vi "Finding_Problem_Dots-3.vi"(3 "error IN":errorcluster, 5 "[IN] Frame-to-frame displ":dbl[][](array[numeric])) -> (0 "error OUT":errorcluster, 2 "[OUT] Dot matrix":i16[][](array[numeric]))   [LabVIEW 2013]
doc: "SubVI searches and highlight the problem displacements for further tracks separation"
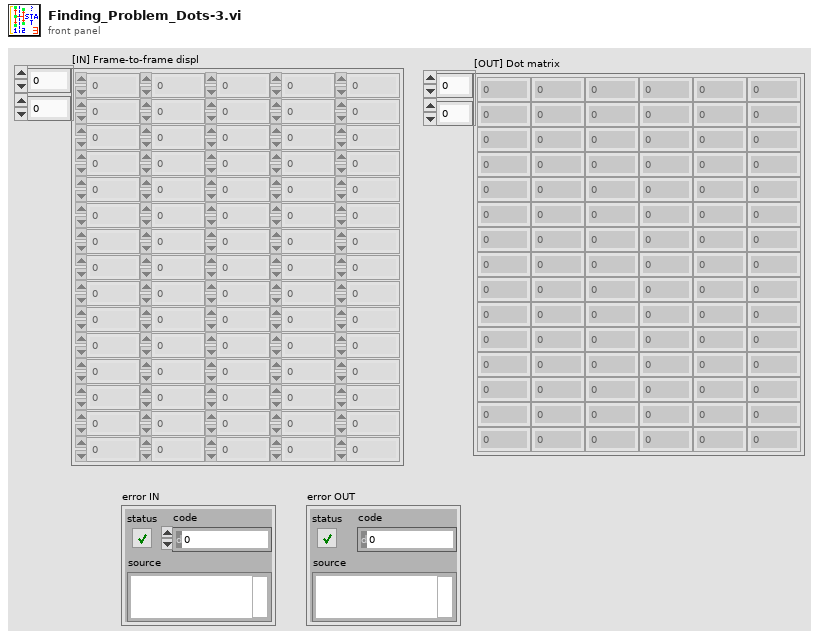
[diagram p1: front panel]
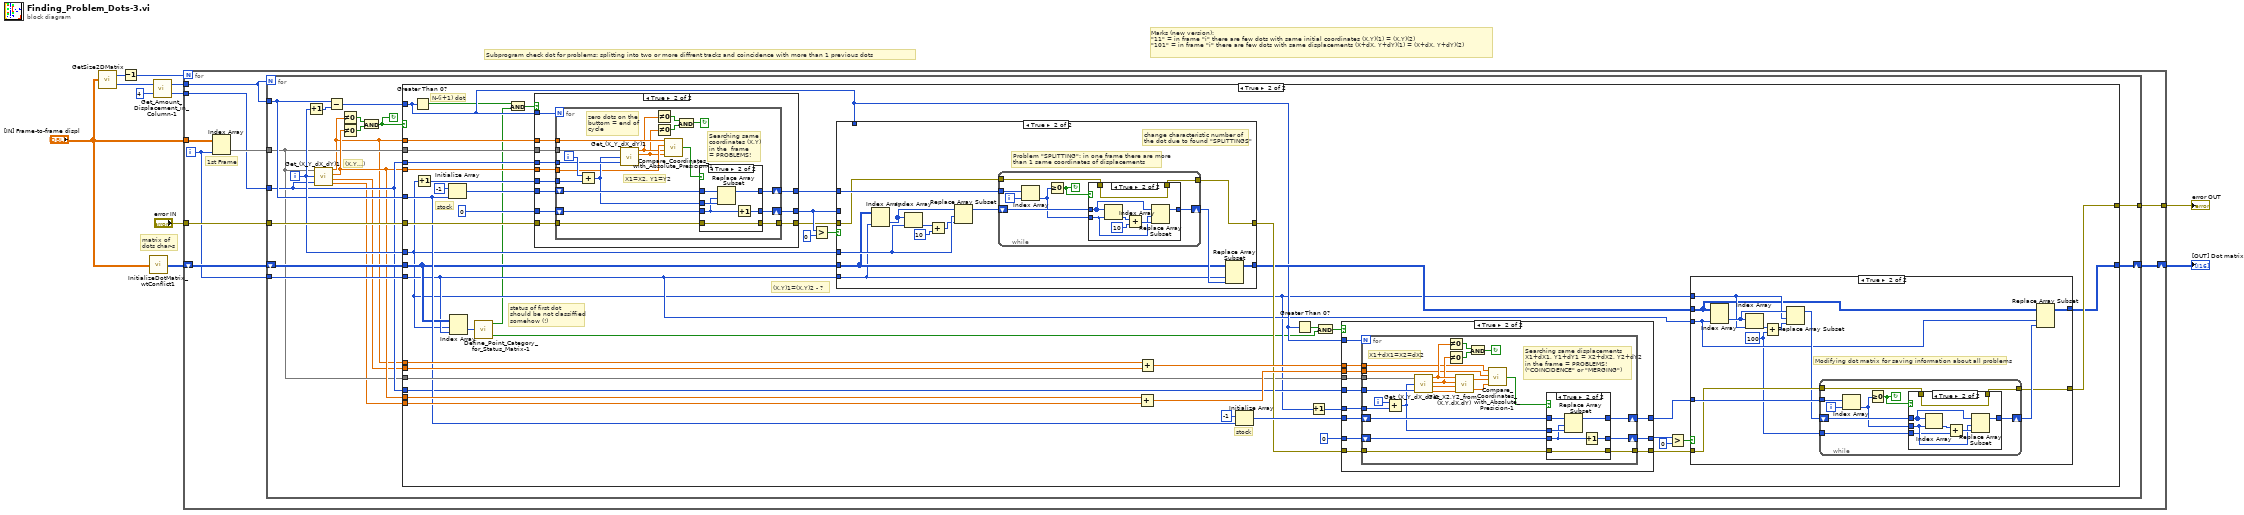
[diagram p0: block diagram]
diagram:
  # "Marks (new version): \n\"11\" = in frame \"i\" there are few dots with same initial coordinates (X,Y)(1) = (X,Y)(2)\n\"101\" = in frame \"i\" there are few dots with same displacements (X+dX, Y+dY)(1) = (X+dX, Y+dY)(2)"
  # "matrix of\ndots char-s"
  # "Subprogram check dot for problems: splitting into two or more diffrent tracks and coincidence with more than 1 previous dots"
  n1 = call "GetSize2DMatrix.vi"("Array IN (2D)"="[IN] Frame-to-frame displ") -> ("# Cols"=w9:i32, "# Rows"=w4:i32)
  n2 = Decrement(x=w9) -> (x-1=w11:i32)
  n3 = call "InitializeDotMatrix_wtConflict1.vi"("Frame-to-frame displ"="[IN] Frame-to-frame displ") -> ("Dot matrix"=w8:i16[][])
  n4 = call "Get_Amount_Displacement_in_Column-1.vi"("multiplier"=4 ("y"), "# Rows"=w4) -> ("multiplier out"=w1:i32, "Displ amount"=w2:i32)
  n5 = for {
    N: w11 -> [_]
    tunnel: "error IN" -> [w20]
    tunnel: [w19] -> w7
    shift-right: [w14] -> w6
    shift-left: w8 -> [w16]
    tunnel: "[IN] Frame-to-frame displ" -> [w17]
    tunnel: w2 -> [w13]
    tunnel: w1 -> [w12]
    i -> [w15]
    # "1st Frame"
    n6 = Index Array(array=w17, index (col)=w15) -> (element=w18:dbl[])  [unwired: 1 in]
    n7 = for {
      N: w13 -> [_]
      tunnel: w12 -> [w26]
      tunnel: w20 -> [w36]
      tunnel: [w35] -> w19
      tunnel: w18 -> [w24]
      tunnel: w13 -> [w30]
      shift-right: [w27] -> w14
      shift-left: w16 -> [w29]
      tunnel: w15 -> [w28]
      i -> [w33]
      stop <- w34 continue-if-true
      # "(X,Y...)"
      n8 = Increment(x=w33) -> (x+1=w32:i32)
      n9 = call "Get_(X_Y_dX_dY)1.vi"("(X,Y,dX,dY)"=w24, "index"=w33, "multiplier"=w26) -> ("X"=w21:dbl, "Y"=w25:dbl, "dX"=w23:dbl, "dY"=w22:dbl)
      n10 = Subtract(x=w30, y=w32) -> (x-y=w31:i32)
      n11 = Not Equal To 0?(x=w21) -> (x != 0?=w38:bool)
      n12 = Not Equal To 0?(x=w25) -> (x != 0?=w37:bool)
      n13 = And(x=w38, y=w37) -> (x .and. y?=w34:bool)
      n14 = case shown="True" w34 {
        tunnel: w21 -> [_ w84]
        tunnel: w25 -> [_ w82]
        tunnel: w36 -> [w40 w77]
        tunnel: [w40 w52] -> w35
        tunnel: w33 -> [_ w46]
        tunnel: w31 -> [_ w60]
        tunnel: w24 -> [_ w85]
        tunnel: w26 -> [_ w83]
        tunnel: w30 -> [_ w54]
        tunnel: w29 -> [w39 w48]
        tunnel: w28 -> [_ w47]
        tunnel: [w39 w51] -> w27
        tunnel: w26 -> [_ w53]
        tunnel: w21 -> [_ w59]
        tunnel: w25 -> [_ w57]
        tunnel: w24 -> [_ w55]
        tunnel: w23 -> [_ w58]
        tunnel: w22 -> [_ w56]
        frame False {
        }
        frame True {
          # "status of first dot\nshould be not classiffied\nsomehow (!)"
          # "stock"
          # "(X,Y)1=(X,Y)2 - ?"
          # "stock"
          # "N-(i+1) dot"
          n15 = Greater Than 0?(x=w60) -> (x > 0?=w50:bool)
          n16 = Increment(x=w46) -> (x+1=w81:i32)
          n17 = Initialize Array(-1 ("element"), w54) -> (w79:i32[])
          n18 = Index Array(array=w48, index (row)=w46, index (col)=w47) -> (element=w45:i16)
          n19 = call "Define_Point_Category_for_Status_Matrix-1.vi"("[IN] Summarized\npoint status"=w45) -> ("[OUT] Point isn't \nlabeled with \"10\""=w44:bool, "[OUT] Point isn't \nlabeled with \"100\""=w41:bool)  [unwired: 1 out]
          n20 = And(x=w50, y=w44) -> (x .and. y?=w49:bool)
          n21 = case shown="True" w49 {
            tunnel: w60 -> [_ w182]
            tunnel: w85 -> [_ w181]
            tunnel: w84 -> [_ w180]
            tunnel: w82 -> [_ w179]
            tunnel: w83 -> [_ w178]
            tunnel: w81 -> [_ w177]
            tunnel: [w170 w176] -> w74
            tunnel: [w169 w175] -> w76
            tunnel: w79 -> [w170 w174]
            tunnel: 0 -> [w169 w173]
            tunnel: w77 -> [w168 w172]
            tunnel: [w168 w171] -> w75
            frame False {
            }
            frame True {
              n22 = for {
                N: w182 -> [_]
                tunnel: w178 -> [w192]
                tunnel: w181 -> [w201]
                tunnel: w180 -> [w186]
                tunnel: w179 -> [w185]
                shift-right: [w196] -> w175
                shift-left: w173 -> [w197]
                tunnel: w177 -> [w194]
                shift-right: [w191] -> w176
                shift-left: w174 -> [w193]
                tunnel: w172 -> [w190]
                tunnel: [w189] -> w171
                i -> [w195]
                stop <- w198 continue-if-true
                # "zero dots on the\nbuttom = end of\ncycle"
                # "X1=X2, Y1=Y2"
                # "Searching same \ncoordinates (X,Y) \nin the  frame \n= PROBLEMS!"
                n23 = Add(x=w195, y=w194) -> (x+y=w188:i32)
                n24 = call "Get_(X_Y_dX_dY)1.vi"("(X,Y,dX,dY)"=w201, "index"=w188, "multiplier"=w192) -> ("X"=w184:dbl, "Y"=w183:dbl)  [unwired: 2 out]
                n25 = Not Equal To 0?(x=w184) -> (x != 0?=w200:bool)
                n26 = Not Equal To 0?(x=w183) -> (x != 0?=w199:bool)
                n27 = call "Compare_Coordinates_with_Absolute_Presicion-1.vi"("X 1"=w186, "Y 1"=w185, "X 2"=w184, "Y 2"=w183) -> ("[OUT] Same coordinates?"=w187:bool)  [unwired: 1 in]
                n28 = And(x=w200, y=w199) -> (x .and. y?=w198:bool)
                n29 = case shown="True" w187 {
                  tunnel: w197 -> [w204 w207]
                  tunnel: [w204 w206] -> w196
                  tunnel: w193 -> [w202 w210]
                  tunnel: w188 -> [_ w209]
                  tunnel: [w202 w208] -> w191
                  tunnel: [w203 w205] -> w189
                  tunnel: w190 -> [w203 w205]
                  frame False {
                  }
                  frame True {
                    n30 = Replace Array Subset(array=w210, new element=w209, index=w207) -> (w208:i32[])
                    n31 = Increment(x=w207) -> (x+1=w206:i32)
                  }
                }
              }
            }
          }
          n32 = Greater?(x=w76, y=0) -> (0:w86:bool)
          n33 = case shown="True" w86 {
            tunnel: w74 -> [_ w224]
            tunnel: w76 -> [_ _]
            tunnel: w75 -> [w212 w217]
            tunnel: w46 -> [_ w225]
            tunnel: [w212 w213] -> w62
            tunnel: w48 -> [w211 w216]
            tunnel: w47 -> [_ w215]
            tunnel: [w211 w214] -> w61
            tunnel: w60 -> [_ _]
            frame False {
            }
            frame True {
              # "change characteristic number of \nthe dot due to found \"SPLITTINGS\""
              # "Problem \"SPLITTING\": in one frame there are more \nthan 1 same coordinates of displacements"
              n34 = Index Array(array=w216, index (col)=w215) -> (element=w223:i16[])  [unwired: 1 in]
              n35 = Index Array(array=w223, index=w225) -> (element=w221:i16)
              n36 = Add(x=w221, y=i16 10) -> (x+y=w219:i16)
              n37 = Replace Array Subset(array=w223, new element=w219, index=w225) -> (w218:i16[])
              n38 = while {
                tunnel: w224 -> [w233]
                shift-right: [w228] -> w222
                shift-left: w218 -> [w230]
                tunnel: w217 -> [w227]
                tunnel: [w226] -> w213
                i -> [w232]
                stop <- w231 continue-if-true
                n39 = Index Array(array=w233, index=w232) -> (element=w229:i32)
                n40 = Greater Or Equal To 0?(x=w229) -> (x >= 0?=w231:bool)
                n41 = case shown="True" w231 {
                  tunnel: w230 -> [w235 w239]
                  tunnel: w229 -> [_ w238]
                  tunnel: [w235 w237] -> w228
                  tunnel: w227 -> [w234 w236]
                  tunnel: [w234 w236] -> w226
                  frame False {
                  }
                  frame True {
                    n42 = Index Array(array=w239, index=w238) -> (element=w241:i16)
                    n43 = Add(x=w241, y=i16 10) -> (x+y=w240:i16)
                    n44 = Replace Array Subset(array=w239, new element=w240, index=w238) -> (w237:i16[])
                  }
                }
              }
              n45 = Replace Array Subset(array=w216, new element=w222, index (col)=w215) -> (w214:i16[][])  [unwired: 1 in]
            }
          }
          n46 = Add(x=w57, y=w56) -> (x+y=w64:dbl)
          n47 = Add(x=w59, y=w58) -> (x+y=w63:dbl)
          n48 = Initialize Array(-1 ("element"), w54) -> (w68:i32[])
          n49 = Greater Than 0?(x=w60) -> (x > 0?=w43:bool)
          n50 = Increment(x=w46) -> (x+1=w65:i32)
          n51 = And(x=w43, y=w41) -> (x .and. y?=w42:bool)
          n52 = case shown="True" w42 {
            tunnel: w60 -> [_ w135]
            tunnel: w55 -> [_ w134]
            tunnel: w63 -> [_ w133]
            tunnel: w64 -> [_ w132]
            tunnel: w53 -> [_ w131]
            tunnel: w65 -> [_ w130]
            tunnel: [w123 w129] -> w73
            tunnel: [w122 w128] -> w70
            tunnel: w68 -> [w123 w127]
            tunnel: 0 -> [w122 w126]
            tunnel: w62 -> [w121 w125]
            tunnel: [w121 w124] -> w72
            frame False {
            }
            frame True {
              n53 = for {
                N: w135 -> [_]
                tunnel: w131 -> [w149]
                tunnel: w134 -> [w158]
                tunnel: w133 -> [w138]
                tunnel: w132 -> [w137]
                shift-right: [w153] -> w128
                shift-left: w126 -> [w154]
                tunnel: w130 -> [w151]
                shift-right: [w148] -> w129
                shift-left: w127 -> [w150]
                tunnel: w125 -> [w147]
                tunnel: [w146] -> w124
                i -> [w152]
                stop <- w155 continue-if-true
                # "X1+dX1=X2=dX2"
                # "Searching same displacements \nX1+dX1, Y1+dY1 = X2+dX2, Y2+dY2\nin the frame = PROBLEMS! (\"COINCIDENCE\" or \"MERGING\")"
                n54 = Add(x=w152, y=w151) -> (x+y=w145:i32)
                n55 = call "Get_(X_Y_dX_dY)1.vi"("(X,Y,dX,dY)"=w158, "index"=w145, "multiplier"=w149) -> ("X"=w144:dbl, "Y"=w143:dbl, "dX"=w142:dbl, "dY"=w141:dbl)
                n56 = Not Equal To 0?(x=w144) -> (x != 0?=w157:bool)
                n57 = Not Equal To 0?(x=w143) -> (x != 0?=w156:bool)
                n58 = call "Get_X2,Y2_from_(X,Y,dX,dY).vi"("dY"=w141, "dX"=w142, "Y1"=w143, "X1"=w144) -> ("Y2 = (Y1+dY)"=w139:dbl, "X2 = (X1+dX)"=w140:dbl)
                n59 = And(x=w157, y=w156) -> (x .and. y?=w155:bool)
                n60 = call "Compare_Coordinates_with_Absolute_Presicion-1.vi"("X 1"=w138, "Y 1"=w137, "X 2"=w140, "Y 2"=w139) -> ("[OUT] Same coordinates?"=w136:bool)  [unwired: 1 in]
                n61 = case shown="True" w136 {
                  tunnel: w154 -> [w161 w164]
                  tunnel: [w161 w163] -> w153
                  tunnel: w150 -> [w159 w167]
                  tunnel: w145 -> [_ w166]
                  tunnel: [w159 w165] -> w148
                  tunnel: [w160 w162] -> w146
                  tunnel: w147 -> [w160 w162]
                  frame False {
                  }
                  frame True {
                    n62 = Replace Array Subset(array=w167, new element=w166, index=w164) -> (w165:i32[])
                    n63 = Increment(x=w164) -> (x+1=w163:i32)
                  }
                }
              }
            }
          }
          n64 = Greater?(x=w70, y=0) -> (0:w71:bool)
          n65 = case shown="True" w71 {
            tunnel: w61 -> [w88 w95]
            tunnel: w47 -> [_ w94]
            tunnel: w46 -> [_ w99]
            tunnel: w72 -> [w89 w97]
            tunnel: w73 -> [_ w98]
            tunnel: [w89 w92] -> w52
            tunnel: [w88 w91] -> w51
            frame False {
            }
            frame True {
              w90 = i16 100 ("y")
              # "Modifying dot matrix for saving information about all problems"
              n66 = Index Array(array=w95, index (col)=w94) -> (element=w100:i16[])  [unwired: 1 in]
              n67 = Index Array(array=w100, index=w99) -> (element=w101:i16)
              n68 = Add(x=w101, y=w90) -> (x+y=w102:i16)
              n69 = Replace Array Subset(array=w100, new element=w102, index=w99) -> (w96:i16[])
              n70 = while {
                tunnel: w98 -> [w111]
                shift-right: [w106] -> w93
                shift-left: w96 -> [w108]
                tunnel: w97 -> [w105]
                tunnel: [w104] -> w92
                tunnel: w90 -> [w103]
                i -> [w110]
                stop <- w109 continue-if-true
                n71 = Index Array(array=w111, index=w110) -> (element=w107:i32)
                n72 = Greater Or Equal To 0?(x=w107) -> (x >= 0?=w109:bool)
                n73 = case shown="True" w109 {
                  tunnel: w108 -> [w113 w118]
                  tunnel: w107 -> [_ w117]
                  tunnel: [w113 w116] -> w106
                  tunnel: w105 -> [w112 w115]
                  tunnel: [w112 w115] -> w104
                  tunnel: w103 -> [_ w114]
                  frame False {
                  }
                  frame True {
                    n74 = Index Array(array=w118, index=w117) -> (element=w120:i16)
                    n75 = Add(x=w120, y=w114) -> (x+y=w119:i16)
                    n76 = Replace Array Subset(array=w118, new element=w119, index=w117) -> (w116:i16[])
                  }
                }
              }
              n77 = Replace Array Subset(array=w95, new element=w93, index (col)=w94) -> (w91:i16[][])  [unwired: 1 in]
            }
          }
        }
      }
    }
  }
  "error OUT" <- w7
  "[OUT] Dot matrix" <- w6
